vi "Create Digital Input and Output Module.vi"   [LabVIEW 2017, in "Scan Engine Scripting.lvlib"]
doc: "Creates and configures an instance of a digital input and output module that can be used to set a slot in a Scan Engine custom device chassis."
uses:
  Scan Engine Scripting.lvlib
  NI 9375/NI 9375.lvclass
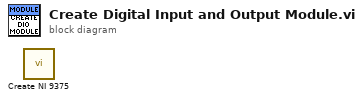
[diagram p0: block diagram]
diagram:
  n1 = call "Create NI 9375.vi"() -> ()  [unwired: 10 in, 2 out]
